vi "Boolean Display thing.vi"() -> ()   [LabVIEW 2018]
panel:
  in  "Sampling Rate (ms)":dbl
  in  "stop":bool
  out "Waveform Chart":T1(graph)
  in  "?":bool
  in  "?":bool
  in  "?":bool
  in  "Line 3":dbl(slide) scale=0.0..10.0
  in  "Line 2":dbl(slide) scale=0.0..10.0
  in  "Line 1":dbl(slide) scale=0.0..10.0
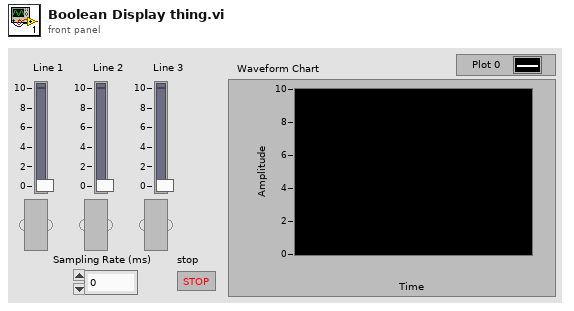
[diagram p1: front panel]
types:
  T1 = cluster{"Line 1":dbl, "Line 2":dbl, "Line 3":dbl}
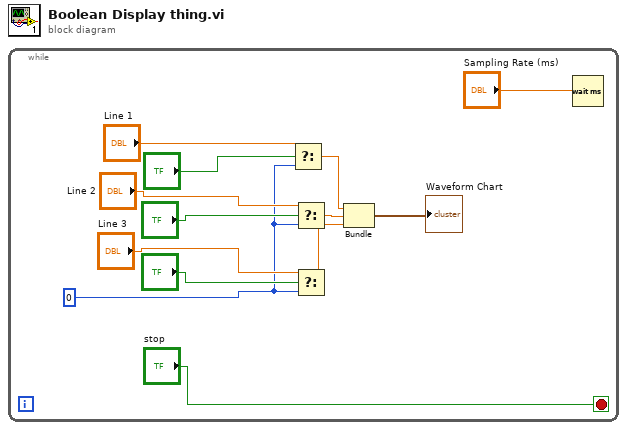
[diagram p0: block diagram]
diagram:
  n1 = while {
    stop <- "stop" stop-if-true
    w3 = 0
    n2 = Select(t="Line 1", s="?", f=w3) -> (s? t:f=w1:dbl)
    n3 = Select(t="Line 2", s="?", f=w3) -> (s? t:f=w12:dbl)
    n4 = Select(t="Line 3", s="?", f=w3) -> (s? t:f=w13:dbl)
    n5 = Bundle("Line 1"=w1, "Line 2"=w12, "Line 3"=w13) -> (→"Waveform Chart":T1)  [unwired: 1 in]
    n6 = Wait (ms)(milliseconds to wait="Sampling Rate (ms)") -> ()  [unwired: 1 out]
  }
